vi "DFD FXP Simulation Report.vi"(8 "error in (no error)":errorcluster, 9 "filtering statistics report":T3(array[cluster]) {"statistical information"."min value" format="%.2f"; "statistical information"."max value" format="%.2f"; "quantizer source" items=["Coefficients a/k"=0, "Coefficients b/v"=7, "Input"=1, "Output"=2, "Multiplicand"=3, "Product"=4, "Sum"=5, "Delay"=6]}) -> (0 "error out":errorcluster, 2 "filtering text report":string)   [LabVIEW 2017, in "NI_DigFilterLicensed.lvlib"]
doc: "Creates a text report of filtering statistics from the DFD FXP Simulation VI or the DFD FXP Simulation with State VI."
uses:
  <vilib>/addons/Digital Filter Design/NI_DigFilterLicensed.lvlib
  <vilib>/addons/Digital Filter Design/_Objects.llb/DFD Quantization Sources.ctl
  <vilib>/addons/Digital Filter Design/_Objects.llb/DFD FXP Statistics Data.ctl
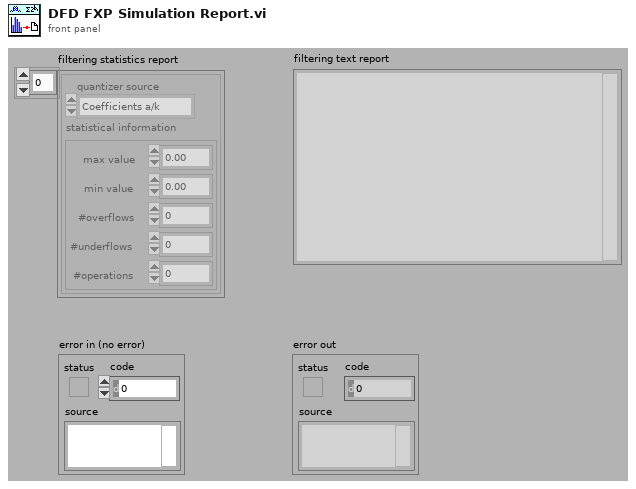
[diagram p1: front panel]
types:
  T1 = typedef "NI_DigFilterLicensed.lvlib/DFD Quantization Sources.ctl" = u16
  T2 = typedef "NI_DigFilterLicensed.lvlib/DFD FXP Statistics Data.ctl" = cluster{"max value":ext, "min value":ext, "#overflows":i32, "#underflows":i32, "#operations":i32}
  T3 = cluster{"quantizer source":T1, "statistical information":T2}[]
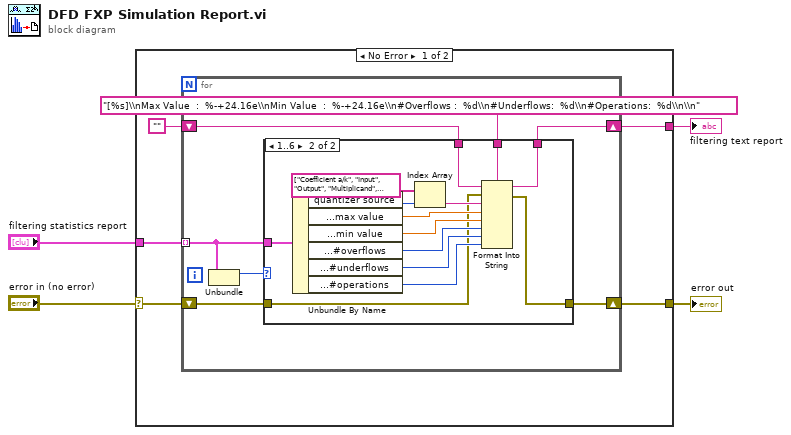
[diagram p0: block diagram]
diagram:
  n1 = case shown="No Error" "error in (no error)" {
    selector: "error in (no error)" -> [w7 w33]
    tunnel: "filtering statistics report" -> [w9 _]
    tunnel: [w8 _] -> w2
    tunnel: [w6 w33] -> w1
    frame No Error {
      n2 = for {
        tunnel: w9 -> [w11] mode=indexing
        shift-right: [w16] -> w8
        shift-left: "" -> [w15]
        shift-right: [w13] -> w6
        shift-left: w7 -> [w14]
        n3 = Unbundle(w11) -> ("quantizer source"=w10:T1)  [unwired: 1 out]
        n4 = case shown="1..6" w10 {
          tunnel: w11 -> [_ w32]
          tunnel: [w18 w23] -> w16
          tunnel: w15 -> [w18 w22]
          tunnel: w14 -> [w17 w21]
          tunnel: [w17 w20] -> w13
          tunnel: "[%s]\\nMax Value  :  %-+24.16e\\nMin Value  :  %-+24.16e\\n#Overflows :  %d\\n#Underflows:  %d\\n#Operations:  %d\\n\\n" ("format string") -> [_ w19]
          frame 0, Default {
          }
          frame 1..6 {
            n5 = Unbundle By Name(w32) -> ("quantizer source"=w31:T1, "statistical information.max value"=w28:ext, "statistical information.min value"=w27:ext, "statistical information.#overflows"=w26:i32, "statistical information.#underflows"=w25:i32, "statistical information.#operations"=w24:i32)
            n6 = Index Array(array=string[] ["Coefficient a/k", "Input", "Output", "Multiplicand", "Product", "Sum", "Delay", "Coefficient b/v"], index=w31) -> (element=w29:string)
            n7 = Format Into String(format string=w19, initial string=w22, error in=w21, w29, w28, w27, w26, w25, w24) -> (resulting string=w23:string, error out=w20:errorcluster)
          }
        }
      }
    }
    frame Error {
    }
  }
  "filtering text report" <- w2
  "error out" <- w1
